vi "Connect Information.vi"(8 "error in (no error)":errorcluster, 10 "Case":string, 11 "CSM-Helper in":refnum<class "CSM-Helper.lvclass">) -> (0 "error out":errorcluster, 1 "Backend Connected Info":T1[](array[typedef]), 2 "FrontEnd Connected Info":T1[](array[typedef]), 3 "CSM-Helper out":refnum<class "CSM-Helper.lvclass">)   [LabVIEW 2020, in "CSM-Helper.lvclass"]
uses:
  CSM-Helper.lvclass
  Typedef/Def-Conncted Information.ctl
  API/Get CaseFrame Reference By CaseName.vi
panel:
  out "Array":string[](array[string])
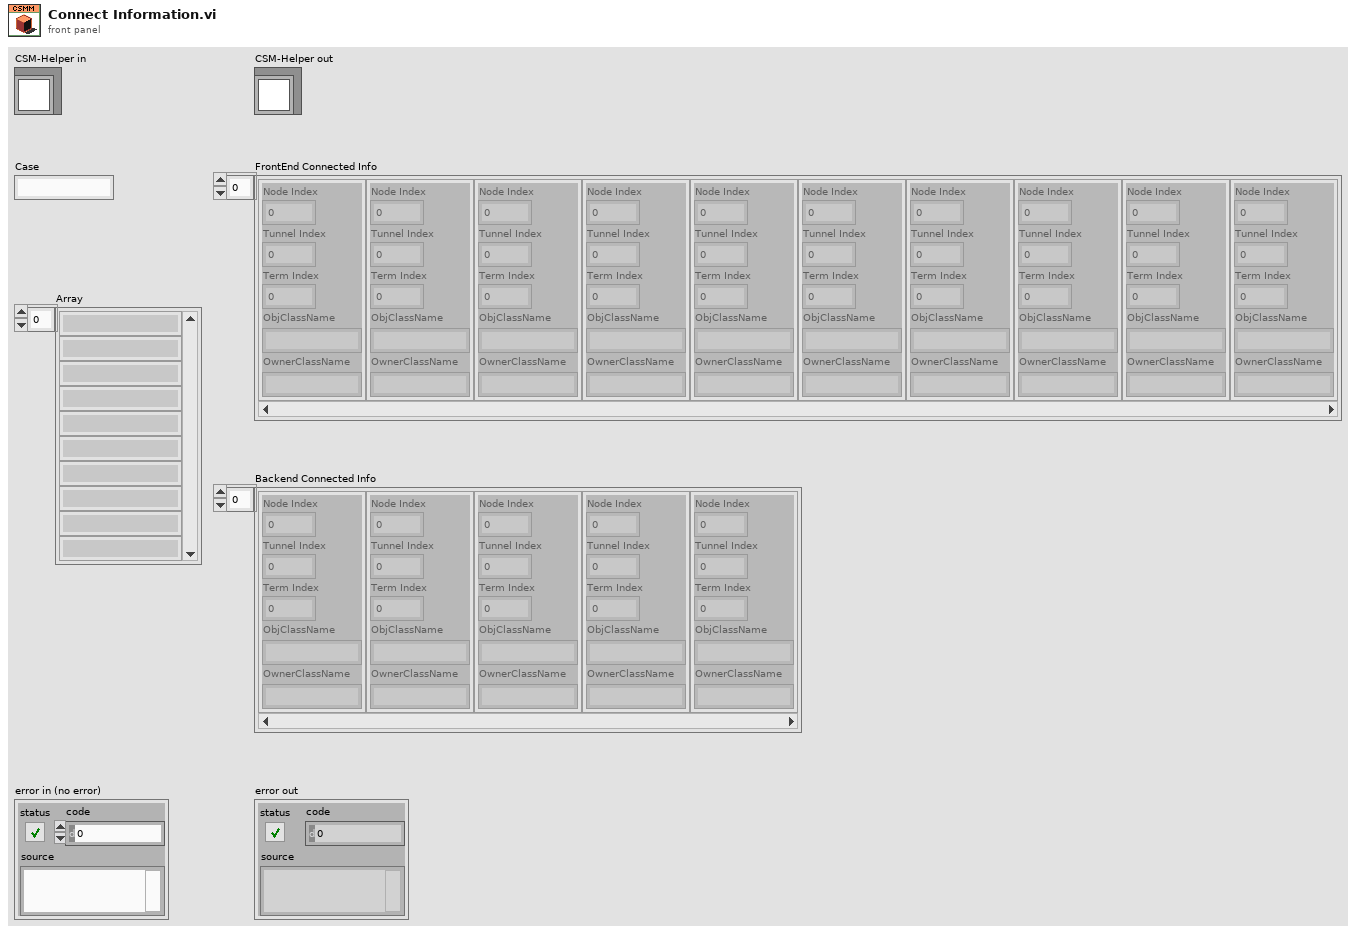
[diagram p1: front panel]
types:
  T1 = typedef "CSM-Helper.lvclass/Def-Conncted Information.ctl" = cluster{"Node Index":i32, "Tunnel Index":i32, "Term Index":i32, "ObjClassName":string, "OwnerClassName":string}
  T2 = cluster{"InternalData":refnum<vi>, "CSM Name":refnum<vi>, "Last Resp":refnum<vi>, "Remaining State":refnum<vi>, "Arguments":refnum<vi>, "Response Source":refnum<vi>, "Source CSM":refnum<vi>, "Selector":refnum<vi>, "Error":refnum<vi>}
  T3 = cluster{"InternalData":refnum<vi>, "Resp":refnum<vi>, "Remaining State":refnum<vi>, "Error":refnum<vi>}
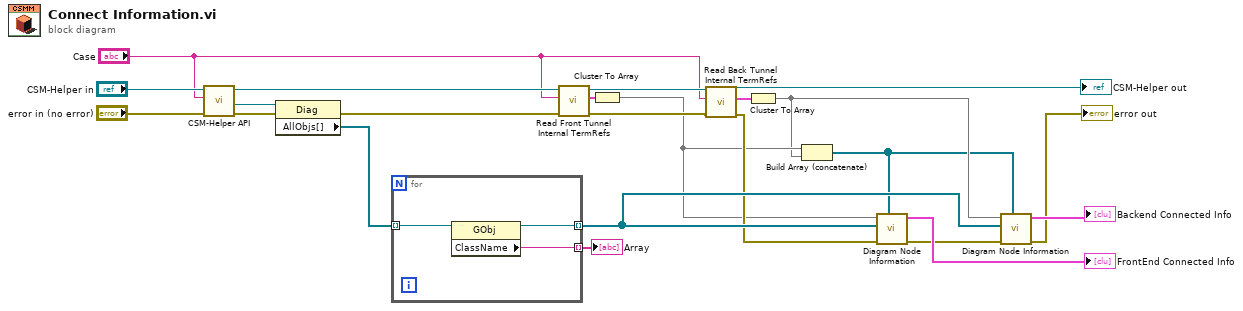
[diagram p0: block diagram]
diagram:
  n1 = call-poly "CSM-Helper API.vi"("error in (no error)"="error in (no error)", "CASE"="Case", "CSM-Helper in"="CSM-Helper in") -> ("error out"=w22:errorcluster, "Frame Refs"=w21:refnum<vi>, "CSM-Helper out"=w19:refnum<class "CSM-Helper.lvclass">)  [unwired: 6 in]
  n2 = property on="Property Node" class="Diag"(reference=w21, error in=w22) -> (error out=w23:errorcluster, "AllObjs[]"=w11:refnum<vi>[])  [unwired: 1 out]
  n3 = for {
    tunnel: [w25] -> w9 mode=indexing
    tunnel: w11 -> [w26] mode=indexing
    tunnel: [w24] -> w10 mode=indexing
    n4 = property class="GObj"(reference=w26) -> (reference out=w25:refnum<vi>, "ClassName"=w24:string)  [unwired: 1 in, 1 out]
  }
  "Array" <- w10
  n5 = call "Read Front Tunnel Internal TermRefs.vi"("error in (no error)"=w23, "case"="Case", "CSM-Helper in"=w19) -> ("error out"=w6:errorcluster, "Front Tunnels"=w15:T2, "CSM-Helper out"=w16:refnum<class "CSM-Helper.lvclass">)  [unwired: 6 in]
  n6 = Cluster To Array(cluster=w15) -> (array=w3:refnum<vi>[])
  n7 = call "Read Back Tunnel Internal TermRefs.vi"("error in (no error)"=w6, "element"="Case", "CSM-Helper in"=w16) -> ("error out"=w4:errorcluster, "Front Tunnels"=w17:T3, "CSM-Helper out"=→"CSM-Helper out":refnum<class "CSM-Helper.lvclass">)  [unwired: 6 in]
  n8 = Cluster To Array(cluster=w17) -> (array=w2:refnum<vi>[])
  n9 = Build Array (concatenate)(w3, w2) -> (w1:refnum<vi>[])
  n10 = call "Diagram Node Information.vi"("InnerTerminal in"=w1, "error in (no error)"=w4, "Array in"=w9, "Front Tunnels"=w3) -> ("error out"=w5:errorcluster, "Array out"=→"FrontEnd Connected Info":T1[])  [unwired: 5 in, 1 out]
  n11 = call "Diagram Node Information.vi"("InnerTerminal in"=w1, "error in (no error)"=w5, "Array in"=w9, "Front Tunnels"=w2) -> ("error out"=→"error out":errorcluster, "Array out"=→"Backend Connected Info":T1[])  [unwired: 5 in, 1 out]
